vi "libssh2_channel_exec.vi"(8 "error in (no error)":errorcluster, 10 "command":string, 11 "Channel":T1) -> (0 "error out":errorcluster, 3 "return value":i32)   [LabVIEW 2013, in "libssh2.lvlib"]
uses:
  libssh2.lvlib
  Channel Refnum.ctl
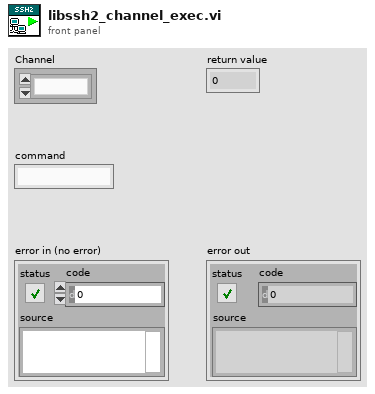
[diagram p1: front panel]
types:
  T1 = typedef "libssh2.lvlib/Channel Refnum.ctl" = refnum<k1>
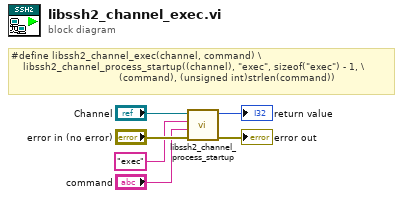
[diagram p0: block diagram]
diagram:
  # "#define libssh2_channel_exec(channel, command) \\\n    libssh2_channel_process_startup((channel), \"exec\", sizeof(\"exec\") - 1, \\\n                                    (command), (unsigned int)strlen(command))"
  n1 = call "libssh2_channel_process_startup.vi"("error in (no error)"="error in (no error)", "message"="command", "request"="exec", "Channel"="Channel") -> ("error out"=→"error out":errorcluster, "return value"=→"return value":i32)  [unwired: 6 in]
